vi "Channel.BuildDisplayedName.vi"(11 "Path":string) -> (3 "Formated Path":string)   [LabVIEW 2015, in "Simple Sequence Tools - Shared.lvlib"]
uses:
  Simple Sequence Tools - Shared.lvlib
  NationalInstruments.VeriStand
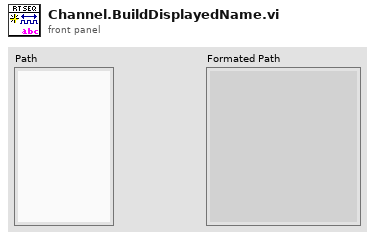
[diagram p1: front panel]
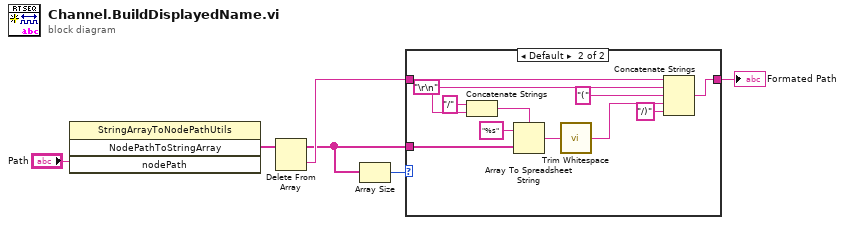
[diagram p0: block diagram]
diagram:
  n1 = invoke class="StringArrayToNodePathUtils" method="NodePathToStringArray"("nodePath"="Path") -> ("NodePathToStringArray"=w4:string[])  [unwired: 3 in, 3 out]
  n2 = Delete From Array(array=w4) -> (deleted portion=w5:string, array with subset deleted=w2:string[])  [unwired: 2 in]
  n3 = Array Size(array=w2) -> (size(s)=w1:i32)
  n4 = case shown="Default" w1 {
    tunnel: w5 -> [w7 w14]
    tunnel: [w7 w9] -> w3
    tunnel: w2 -> [_ w8]
    frame 0 {
    }
    frame Default {
      w17 = "\r\n"
      n5 = Concatenate Strings("/" ("string"), w17) -> (w16:string)
      n6 = Array To Spreadsheet String(delimiter (Tab)=w16, array=w8, 3:"%s" ("format string")) -> (spreadsheet string=w13:string)
      n7 = call <vilib>:"Trim Whitespace.vi"("string"=w13) -> ("trimmed string"=w11:string)  [unwired: 1 in]
      n8 = Concatenate Strings(w14, w17, "(" ("string"), w11, "/)" ("string")) -> (w9:string)
    }
  }
  "Formated Path" <- w3
